vi "(SubVI)I2C_8Bit-8Bit_Read_Array.vi"(5 "Log Ref":refnum<vi>, 7 "Clock":T2=enum."400kHz", 8 "error in (no error)":errorcluster caption="에러 입력(에러 없음)", 9 "Address to Read":T1[](array[typedef]) {"Address" format="%02x"; "Delay(ms)" format="%02x"}, 11 "ID":u8) -> (0 "error out":errorcluster caption="에러 출력", 2 "Log out":string, 3 "Read Data":u8[](array[numeric]) format="%02x")   [LabVIEW 2020]
uses:
  Controls/(Ctrl)I2C_Clock.ctl
  Controls/(Ctrl)I2C_8Bit_Read Array.ctl
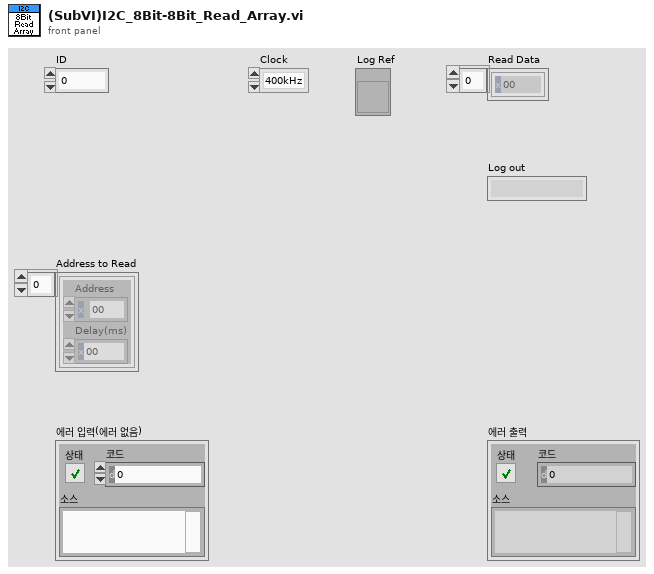
[diagram p1: front panel]
types:
  T1 = typedef "(Ctrl)I2C_8Bit_Read Array.ctl" = cluster{"Address":u8, "Delay(ms)":i32}
  T2 = typedef "(Ctrl)I2C_Clock.ctl" = enum8{"1MHz", "2MHz", "3MHz", "400kHz"}
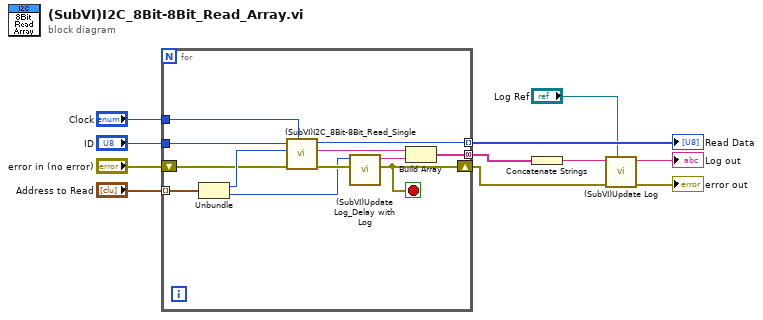
[diagram p0: block diagram]
diagram:
  n1 = for {
    tunnel: "Clock" -> [w23]
    tunnel: "ID" -> [w22]
    tunnel: "Address to Read" -> [w21] mode=indexing
    shift-right: [w17] -> w3
    shift-left: "error in (no error)" -> [w18]
    tunnel: [w15] -> w7 mode=indexing
    tunnel: [w12] -> w6 mode=concatenating
    stop <- w17 stop-if-true
    n2 = Unbundle(w21) -> ("Address"=w20:u8, "Delay(ms)"=w16:i32)
    n3 = call "(SubVI)I2C_8Bit-8Bit_Read_Single.vi"("Clock"=w23, "error in (no error)"=w18, "Address"=w20, "ID"=w22) -> ("error out"=w19:errorcluster, "Log"=w14:string, "Read Data"=w15:u8)  [unwired: 5 in]
    n4 = call "(SubVI)Update Log_Delay with Log.vi"("error in (no error)"=w19, "Delay (ms)"=w16) -> ("error out"=w17:errorcluster, "Log"=w13:string)  [unwired: 8 in]
    n5 = Build Array(w14, w13) -> (w12:string[])
  }
  "Read Data" <- w7
  n6 = Concatenate Strings(w6) -> (w5:string)
  n7 = call "(SubVI)Update Log.vi"("Log Ref"="Log Ref", "error in (no error)"=w3, "Log"=w5) -> ("error out"=→"error out":errorcluster, "Log out"=→"Log out":string)  [unwired: 7 in]
